vi "global path.vi"() -> ()   [LabVIEW 2022 SP3]
panel:
  out "motor status":path=path "membra/motor/support.motor"
  out "fgv list":path=path "membra/fgv lib"
  out "fgv":path=path "membra/fgv"
  out "fgv lib":path=path "membra/fgv lib"
  in  "Framework":u16(ring) items=["Vitruvio", "Local"]
  out "Remote?":bool=TRUE
  out "dock in":path=path "results/dock in"
  out "dock out":path=path "results/dock out"
  in  "whoami":string
  # "Membra"
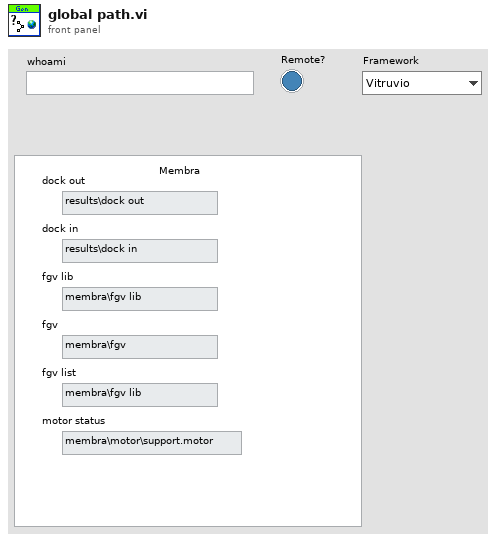
[diagram p1: front panel]
diagram:
